vi "EventLoop.UDP.vi"(0 "Ctrls":refnum<vi>[](array[refnum]), 1 "Name":string, 2 "Path":path) -> ()   [LabVIEW 2014]
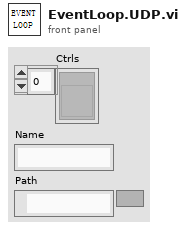
[diagram p1: front panel]
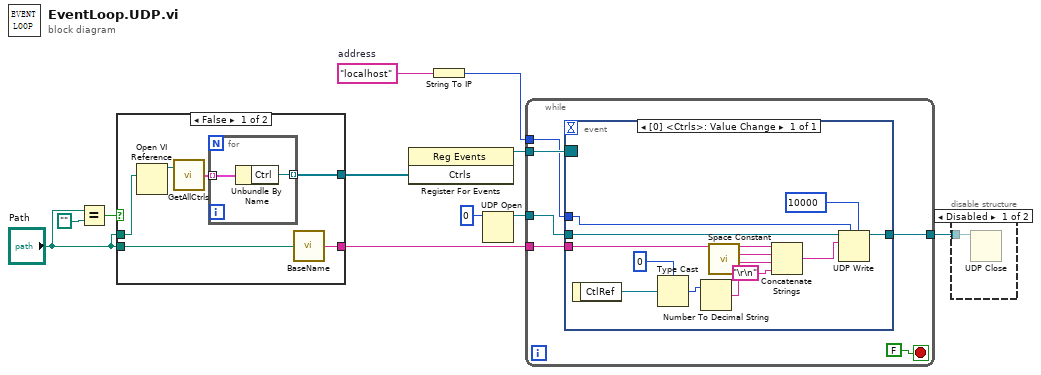
[diagram p0: block diagram]
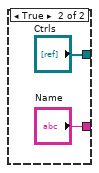
[diagram p2: hidden frame]
diagram:
  w3 = "localhost"  # address
  n1 = Equal?(x="Path", y=path "") -> (x = y?=w8:bool)
  n2 = case shown="False" w8 {
    tunnel: [w14 "Ctrls"] -> w7
    tunnel: [w13 "Name"] -> w4
    tunnel: "Path" -> [w15 _]
    tunnel: "Path" -> [w12 _]
    frame False {
      n3 = Open VI Reference(vi path=w15) -> (vi reference=w16:refnum<vi>)  [unwired: 5 in, 1 out]
      n4 = call "GetAllCtrls.vi"("VI"=w16) -> ("Ctrls"=w17:cluster{"Name":string, "Ctrl":refnum<vi>}[])  [unwired: 1 in]
      n5 = for {
        tunnel: w17 -> [w19] mode=indexing
        tunnel: [w18] -> w14 mode=indexing
        n6 = Unbundle By Name(w19) -> ("Ctrl"=w18:refnum<vi>)
      }
      n7 = call "BaseName.vi"("Path"=w12) -> ("Name"=w13:string)
    }
    frame True {
    }
  }
  n8 = register-events(w7) -> (reference out=w11:refnum<event-registration>)  [unwired: 2 in, 1 out]
  n9 = String To IP(1:w3) -> (0:w2:u32)
  n10 = UDP Open(11:u16 0 ("port")) -> (port=w5:refnum<k16>)  [unwired: 4 in, 2 out]
  n11 = while {
    tunnel: w5 -> [w26]
    tunnel: w11 -> [w25]
    tunnel: [w24] -> w10
    tunnel: w4 -> [w23]
    tunnel: w2 -> [w22]
    stop <- FALSE stop-if-true
    n12 = event shown="[0] <Ctrls>: Value Change" {
      selector: w25 -> [_]
      dyn-events: _ -> [_]
      timeout: _ -> [_]
      tunnel: w26 -> [w31]
      tunnel: [w28] -> w24
      tunnel: w23 -> [w35]
      tunnel: w22 -> [w30]
      event Value Change {
        n13 = event-data() -> ("CtlRef"=w37:refnum<vi>)  [unwired: 1 in]
        n14 = Type Cast(type=u32 0, x=w37) -> (*(type *) &x=w38:u32)
        n15 = Number To Decimal String(number=w38) -> (decimal integer string=w36:string)  [unwired: 1 in]
        n16 = call <vilib>:"Space Constant.vi"() -> ("String"=w33:string)
        n17 = Concatenate Strings(w35, w33, w36, "\r\n") -> (w32:string)
        n18 = UDP Write(address=w30, port or service name=u16 10000, connection ID=w31, data in=w32) -> (3:w28:refnum<k16>)  [unwired: 2 in, 1 out]
      }
    }
  }
  n19 = disable-structure shown="Disabled" {
    disable-tunnel: w10 -> [w40 _]
    frame Disabled {
      n20 = UDP Close(connection ID=w40) -> ()  [unwired: 1 in, 2 out]
    }
    frame Enabled {
    }
  }
